vi "sub_hypot.vi"(10 "dy":dbl, 11 "dx":dbl) -> (3 "length":dbl)   [LabVIEW 2019]
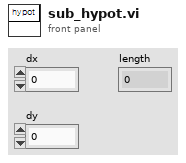
[diagram p1: front panel]
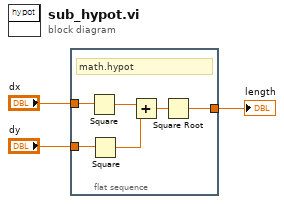
[diagram p0: block diagram]
diagram:
  n1 = flat-sequence {
    tunnel: "dy" -> [w9]
    tunnel: "dx" -> [w8]
    tunnel: [w4] -> w3
    frame #0 {
      # "math.hypot"
      n2 = Square(x=w8) -> (x^2=w6:dbl)
      n3 = Square(x=w9) -> (x^2=w5:dbl)
      n4 = Add(x=w6, y=w5) -> (x+y=w7:dbl)
      n5 = Square Root(x=w7) -> (sqrt(x)=w4:dbl)
    }
  }
  "length" <- w3
